vi "read_raw_dataV2.0.vi"() -> ()   [LabVIEW 2017]
uses:
  <vilib>/Utility/file.llb/Read Delimited Spreadsheet (I64).vi
  <vilib>/Utility/file.llb/Write Delimited Spreadsheet (DBL).vi
  <vilib>/Utility/file.llb/Write Delimited Spreadsheet (I64).vi
  <vilib>/Utility/file.llb/Write Delimited Spreadsheet (string).vi
panel:
  in  "col":i32
  in  "file path (dialog if empty)":path=path "G:/tdc/2017/code_density_rom.mem"
  out "size(s)":i32[](array[numeric])=[2048, 128]
  out "Array":u32[][](array[numeric]) format="%x"
  out "cal":u32[][](graph)
  out "x/y":dbl=0.0025
  out "index":i32=556
  out "time":dbl=31675062850000.0 format="%.000f"
  in  "通道数量":i32=128
  out "fine":u64=861 format="%x"
  out "data 5":string
  in  "ch list":u16[](array[numeric])=[0, 1, 2, 3, 4, 5, 6, 7]
  in  "codeDensity":path=path "G:/tdc/2017/test_20240607_060014_codeDensity.csv"
  out "file path (dialog if empty) 2":path=path "G:/tdc/2017/test_20240327_022214.txt"
  out "ip":u64=35 format="%x"
  out "data 9":string="#"
  out "result string":string="test_20240327_022214"
  out "sent number":u64=71 format="%x"
  out "trigger number":u64=71 format="%x"
  out "data 8":string
  out "data 7":string
  out "data":u64[](array[numeric])=[35, 5, 71, 71, 31675062850000] format="%x"
  out "data 2":string
  out "data 4":string
  out "coarse time":u64=12670025140 format="%x"
  out "error out":errorcluster
  out "substring":string="…"
  out "number 3":u32
  out "channel number":u64=5 format="%x"
  in  "channel":u64
  out "data 6":string
  out "data 3":string="Z"
  in  "dat file (use dialog)":path=path "G:/tdc/2017/test_20240607_060014.dat"
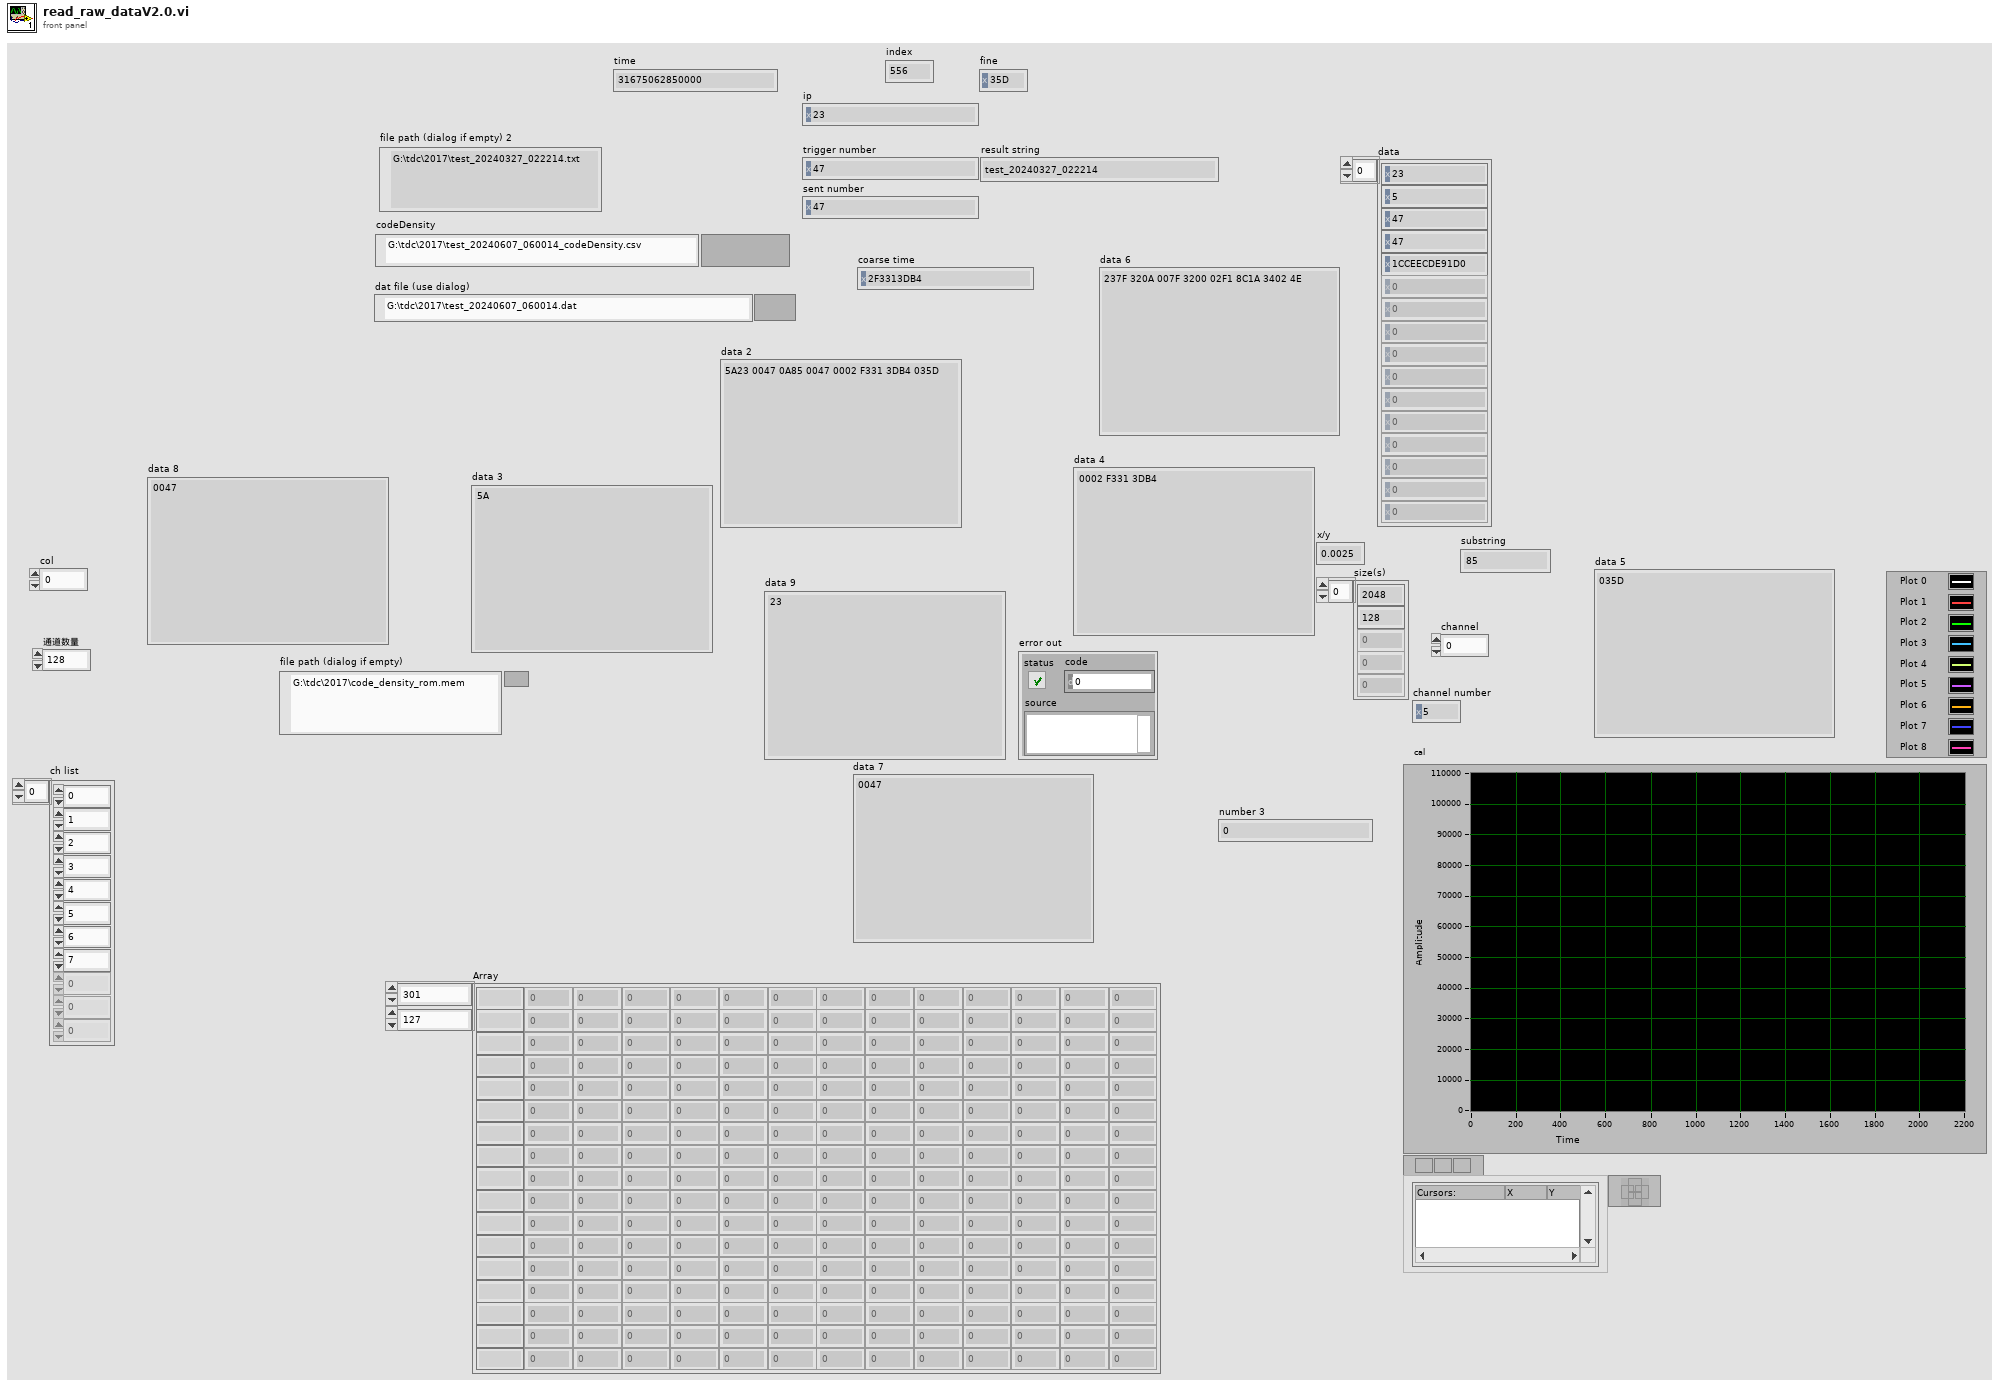
[diagram p1: front panel]
types:
  T1 = enum16{"open", "replace", "create", "open or create", "replace or create", "replace or create with confirmation"}
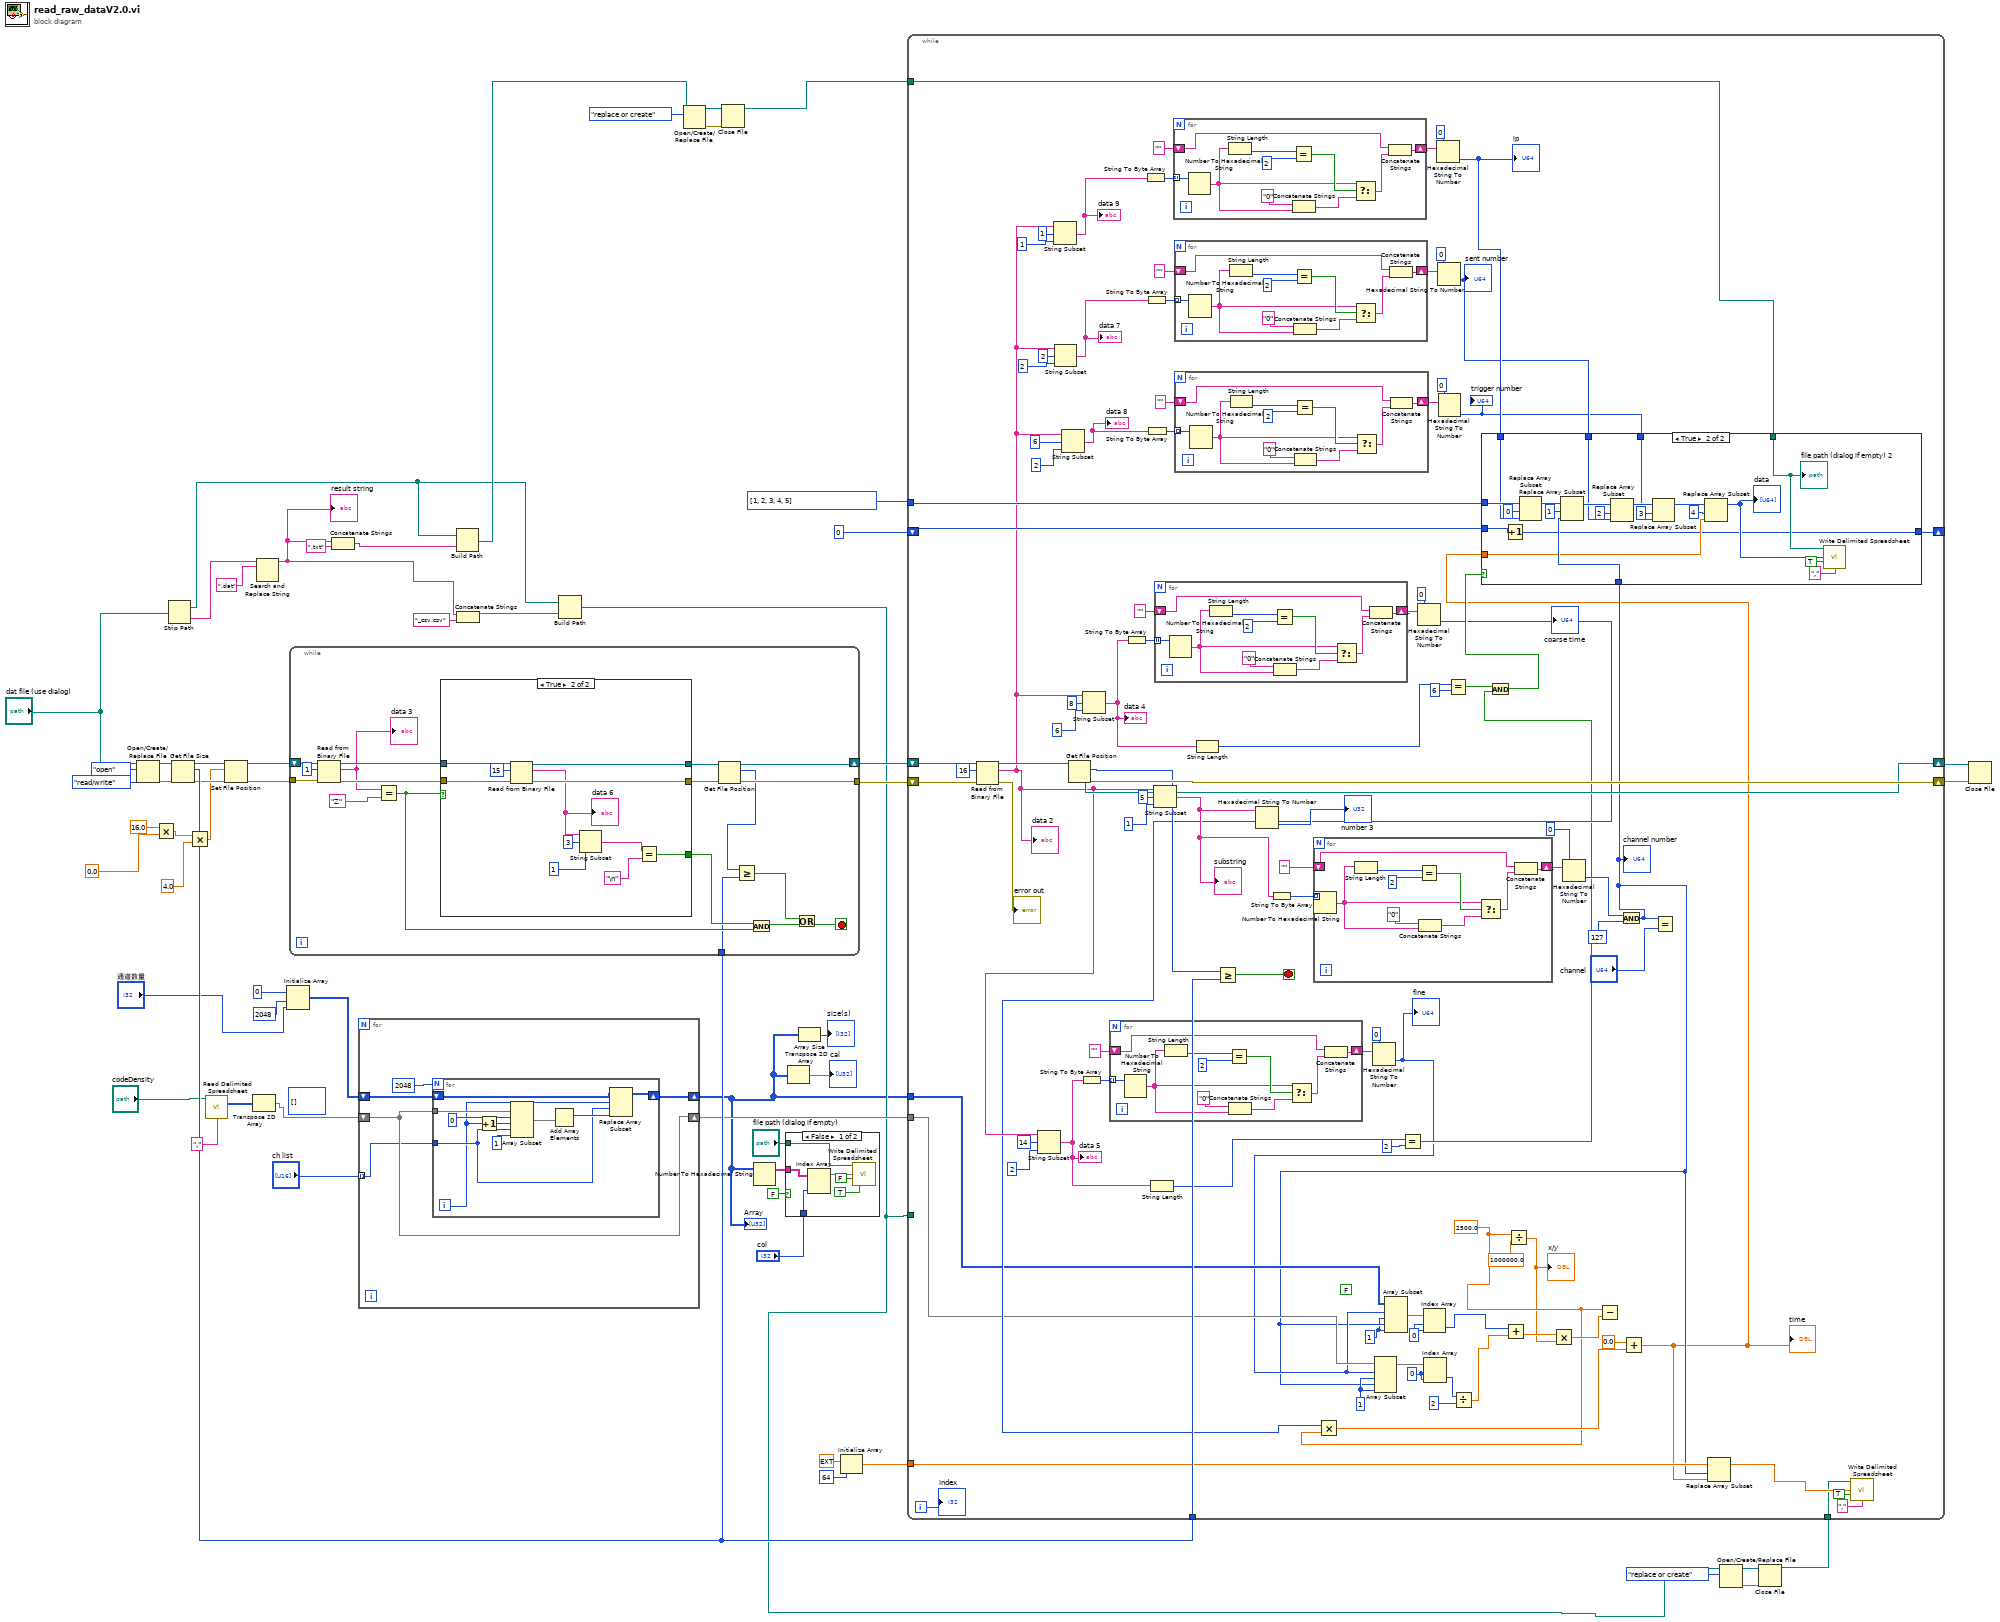
[diagram p0: block diagram]
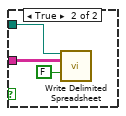
[diagram p2: hidden frame]
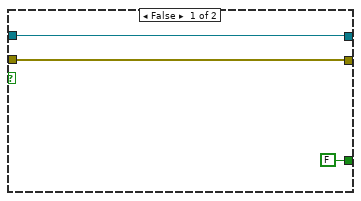
[diagram p4: hidden frame]
diagram:
  (unwired) i64[][] []
  n1 = Open/Create/Replace File(file path (use dialog)="dat file (use dialog)", operation (0:open)=T1."open", access (0:read/write)=enum16{"read/write", "read-only", "write-only"}."read/write") -> (refnum out=w59:refnum<file>, error out=w54:errorcluster)  [unwired: 3 in, 1 out]
  n2 = Multiply(x=16.0, y=0.0) -> (x*y=w20:dbl)
  n3 = Strip Path(path="dat file (use dialog)") -> (stripped path=w9:path, name=w47:string)
  n4 = Get File Size(file=w59, error in=w54) -> (refnum out=w26:refnum<file>, size (in bytes)=w49:i64, 0:w24:errorcluster)
  n5 = Multiply(x=w20, y=4.0) -> (x*y=w18:dbl)
  n6 = call-poly <vilib>:"Read Delimited Spreadsheet.vi"("file path (dialog if empty)"="codeDensity", "delimiter (\\t)"="," ("delimiter (\\t)")) -> ("all rows"=w43:i64[][])  [unwired: 8 in, 5 out]
  n7 = Set File Position(offset (in bytes) (0)=w18, refnum=w26, error in=w24) -> (refnum out=w25:refnum<file>, error out=w23:errorcluster)  [unwired: 1 in]
  n8 = Transpose 2D Array(2D array=w43) -> (transposed array=w31:i64[][])
  n9 = Search and Replace String(input string=w47, search string=".dat") -> (result string=w11:string)  [unwired: 6 in, 3 out]
  "result string" <- w11
  n10 = Initialize Array(u32 0 ("element"), 2048 ("dimension size"), "通道数量") -> (w32:u32[][])
  n11 = while {
    tunnel: w23 -> [w76]
    shift-right: [w64] -> w55
    shift-left: w25 -> [w77]
    tunnel: [w65] -> w56
    tunnel: w49 -> [w63]
    stop <- w61 stop-if-true
    n12 = Read from Binary File(8:w76, 10:1 ("count (1)"), 11:w77) -> (0:w72:errorcluster, 2:w70:string, 3:w73:refnum<file>)  [unwired: 3 in, 1 out]
    "data 3" <- w70
    n13 = Equal?(x=w70, y="Z") -> (x = y?=w67:bool)
    n14 = case shown="True" w67 {
      tunnel: w73 -> [w80 w91]
      tunnel: w72 -> [w79 w90]
      tunnel: [w80 w88] -> w71
      tunnel: [w79 w87] -> w66
      tunnel: [FALSE w81] -> w68
      frame False {
      }
      frame True {
        n15 = Read from Binary File(8:w90, 10:15 ("count (1)"), 11:w91) -> (0:w87:errorcluster, 2:w84:string, 3:w88:refnum<file>)  [unwired: 3 in, 1 out]
        "data 6" <- w84
        n16 = String Subset(string=w84, offset (0)=3, length (rest)=1 ("length (rest)")) -> (substring=w83:string)
        n17 = Equal?(x=w83, y="\n") -> (x = y?=w81:bool)
      }
    }
    n18 = Get File Position(4:w66, 7:w71) -> (0:w65:errorcluster, 2:w62:i64, 3:w64:refnum<file>)
    n19 = Greater Or Equal?(x=w62, y=w63) -> (x >= y?=w60:bool)
    n20 = Compound Arithmetic op=AND(w68, w67) -> (w69:bool)
    n21 = Or(x=w60, y=w69) -> (x .or. y?=w61:bool)
  }
  n22 = Concatenate Strings(w11, ".txt" ("string")) -> (w44:string)
  n23 = for {
    shift-right: [w94] -> w4
    shift-left: w32 -> [w95]
    shift-right: [w93] -> w39
    shift-left: w31 -> [w93]
    tunnel: "ch list" -> [w92] mode=indexing
    n24 = for {
      N: 2048 -> [_]
      tunnel: w93 -> [w106]
      tunnel: w92 -> [w99]
      shift-right: [w101] -> w94
      shift-left: w95 -> [w102]
      i -> [w98]
      n25 = Increment(x=w98) -> (x+1=w97:i32)
      n26 = Array Subset(array=w106, index (row)=0 ("索引"), length (row)=w97, index (col)=w99, length (col)=1 ("长度")) -> (w103:i64[][])
      n27 = Add Array Elements(numeric array=w103) -> (sum=w100:i64)
      n28 = Replace Array Subset(array=w102, new element=w100, index (row)=w98, index (col)=w99) -> (w101:u32[][])
    }
  }
  "Array" <- w4
  n29 = Build Path(base path=w9, name or relative path=w44) -> (appended path=w14:path)
  n30 = Concatenate Strings(w11, "_csv.csv" ("string")) -> (w10:string)
  n31 = Build Path(base path=w9, name or relative path=w10) -> (appended path=w8:path)
  n32 = Open/Create/Replace File(file path (use dialog)=w14, operation (0:open)=T1."replace or create") -> (refnum out=w15:refnum<file>, error out=w16:errorcluster)  [unwired: 4 in, 1 out]
  n33 = Close File(refnum=w15, error in=w16) -> (path=w13:path)  [unwired: 1 out]
  n34 = Number To Hexadecimal String(2:w4) -> (0:w3:string[][])  [unwired: 1 in]
  n35 = case shown="False" FALSE {
    tunnel: "file path (dialog if empty)" -> [w111 w115]
    tunnel: w3 -> [w110 w113]
    tunnel: "col" -> [w108 _]
    frame False {
      n36 = Index Array(array=w110, index (col)=w108) -> (element=w109:string[])  [unwired: 1 in]
      n37 = call-poly <vilib>:"Write Delimited Spreadsheet.vi"("file path (dialog if empty)"=w111, "1D data"=w109, "append to file? (new file:F)"=FALSE, "transpose? (no:F)"=TRUE) -> ()  [unwired: 10 in, 2 out]
    }
    frame True {
      n38 = call-poly <vilib>:"Write Delimited Spreadsheet.vi"("file path (dialog if empty)"=w115, "2D data"=w113, "append to file? (new file:F)"=FALSE) -> ()  [unwired: 11 in, 2 out]
    }
  }
  n39 = Transpose 2D Array(2D array=w4) -> (transposed array=→"cal":u32[][])
  n40 = Array Size(array=w4) -> (size(s)=→"size(s)":i32[])
  n41 = Initialize Array(ext 0.0 ("element"), 64 ("dimension size")) -> (w36:ext[])
  n42 = Open/Create/Replace File(file path (use dialog)=w8, operation (0:open)=T1."replace or create") -> (refnum out=w28:refnum<file>, error out=w29:errorcluster)  [unwired: 4 in, 1 out]
  n43 = Close File(refnum=w28, error in=w29) -> (path=w27:path)  [unwired: 1 out]
  n44 = while {
    shift-right: [w210] -> w53
    shift-left: w55 -> [w214]
    shift-right: [w212] -> w52
    shift-left: w56 -> [w215]
    tunnel: w49 -> [w208]
    shift-right: [w156] -> _
    shift-left: 0 ("length (rest)") -> [w187]
    tunnel: w13 -> [w157]
    tunnel: u64[] [1, 2, 3, 4, 5] -> [w186]
    tunnel: w4 -> [w130]
    tunnel: w39 -> [w131]
    tunnel: w36 -> [w126]
    tunnel: w27 -> [w118]
    tunnel: w8 -> [_]
    i -> [w117]
    stop <- w207 stop-if-true
    w119 = 0 ("index (row)")
    w121 = 1 ("长度")
    w133 = 2500.0 ("x")
    (unwired) FALSE
    w147 = 0 ("索引 (行)")
    w149 = 1 ("长度")
    n45 = Read from Binary File(8:w215, 10:16 ("count (1)"), 11:w214) -> (0:→"error out":errorcluster, 2:w135:string, 3:w211:refnum<file>)  [unwired: 3 in, 1 out]
    "data 2" <- w135
    n46 = String Subset(string=w135, offset (0)=14, length (rest)=2 ("length (rest)")) -> (substring=w138:string)
    "data 5" <- w138
    n47 = String Subset(string=w135, offset (0)=1, length (rest)=1 ("length (rest)")) -> (substring=w167:string)
    "data 9" <- w167
    n48 = String Subset(string=w135, offset (0)=2, length (rest)=2 ("length (rest)")) -> (substring=w168:string)
    "data 7" <- w168
    n49 = String Subset(string=w135, offset (0)=6, length (rest)=2 ("length (rest)")) -> (substring=w173:string)
    "data 8" <- w173
    n50 = Get File Position(7:w211) -> (0:w212:errorcluster, 2:w209:i64, 3:w210:refnum<file>)  [unwired: 1 in]
    n51 = String To Byte Array(string=w138) -> (unsigned byte array=w141:u8[])
    n52 = String Subset(string=w135, offset (0)=8, length (rest)=6 ("length (rest)")) -> (substring=w184:string)
    "data 4" <- w184
    n53 = for {
      shift-right: [w224] -> w140
      shift-left: "" ("format string") -> [w221]
      tunnel: w141 -> [w225] mode=indexing
      n54 = Number To Hexadecimal String(2:w225) -> (0:w217:string)  [unwired: 1 in]
      n55 = String Length(string=w217) -> (length=w223:i32)
      n56 = Equal?(x=w223, y=2) -> (x = y?=w220:bool)
      n57 = Concatenate Strings("0" ("format string"), w217) -> (w219:string)
      n58 = Select(t=w217, s=w220, f=w219) -> (s? t:f=w216:string)
      n59 = Concatenate Strings(w221, w216) -> (w224:string)
    }
    n60 = String To Byte Array(string=w184) -> (unsigned byte array=w203:u8[])
    n61 = String To Byte Array(string=w167) -> (unsigned byte array=w164:u8[])
    n62 = String To Byte Array(string=w168) -> (unsigned byte array=w171:u8[])
    n63 = String To Byte Array(string=w173) -> (unsigned byte array=w175:u8[])
    n64 = String Length(string=w138) -> (length=w137:i32)
    n65 = String Subset(string=w135, offset (0)=5, length (rest)=1 ("length (rest)")) -> (substring=w190:string)
    "substring" <- w190
    n66 = for {
      shift-right: [w296] -> w202
      shift-left: "" ("format string") -> [w293]
      tunnel: w203 -> [w297] mode=indexing
      n67 = Number To Hexadecimal String(2:w297) -> (0:w289:string)  [unwired: 1 in]
      n68 = String Length(string=w289) -> (length=w295:i32)
      n69 = Equal?(x=w295, y=2) -> (x = y?=w292:bool)
      n70 = Concatenate Strings("0" ("format string"), w289) -> (w291:string)
      n71 = Select(t=w289, s=w292, f=w291) -> (s? t:f=w288:string)
      n72 = Concatenate Strings(w293, w288) -> (w296:string)
    }
    n73 = for {
      shift-right: [w234] -> w165
      shift-left: "" ("format string") -> [w231]
      tunnel: w164 -> [w235] mode=indexing
      n74 = Number To Hexadecimal String(2:w235) -> (0:w227:string)  [unwired: 1 in]
      n75 = String Length(string=w227) -> (length=w233:i32)
      n76 = Equal?(x=w233, y=2) -> (x = y?=w230:bool)
      n77 = Concatenate Strings("0" ("format string"), w227) -> (w229:string)
      n78 = Select(t=w227, s=w230, f=w229) -> (s? t:f=w226:string)
      n79 = Concatenate Strings(w231, w226) -> (w234:string)
    }
    n80 = for {
      shift-right: [w244] -> w170
      shift-left: "" ("format string") -> [w241]
      tunnel: w171 -> [w245] mode=indexing
      n81 = Number To Hexadecimal String(2:w245) -> (0:w237:string)  [unwired: 1 in]
      n82 = String Length(string=w237) -> (length=w243:i32)
      n83 = Equal?(x=w243, y=2) -> (x = y?=w240:bool)
      n84 = Concatenate Strings("0" ("format string"), w237) -> (w239:string)
      n85 = Select(t=w237, s=w240, f=w239) -> (s? t:f=w236:string)
      n86 = Concatenate Strings(w241, w236) -> (w244:string)
    }
    n87 = for {
      shift-right: [w254] -> w176
      shift-left: "" ("format string") -> [w251]
      tunnel: w175 -> [w255] mode=indexing
      n88 = Number To Hexadecimal String(2:w255) -> (0:w247:string)  [unwired: 1 in]
      n89 = String Length(string=w247) -> (length=w253:i32)
      n90 = Equal?(x=w253, y=2) -> (x = y?=w250:bool)
      n91 = Concatenate Strings("0" ("format string"), w247) -> (w249:string)
      n92 = Select(t=w247, s=w250, f=w249) -> (s? t:f=w246:string)
      n93 = Concatenate Strings(w251, w246) -> (w254:string)
    }
    n94 = String Length(string=w184) -> (length=w182:i32)
    n95 = Greater Or Equal?(x=w209, y=w208) -> (x >= y?=w207:bool)
    n96 = Hexadecimal String To Number(string=w190) -> (number=→"number 3":u32)  [unwired: 2 in, 1 out]
    n97 = String To Byte Array(string=w190) -> (unsigned byte array=w193:u8[])
    n98 = for {
      shift-right: [w286] -> w192
      shift-left: "" ("format string") -> [w283]
      tunnel: w193 -> [w287] mode=indexing
      n99 = Number To Hexadecimal String(2:w287) -> (0:w279:string)  [unwired: 1 in]
      n100 = String Length(string=w279) -> (length=w285:i32)
      n101 = Equal?(x=w285, y=2) -> (x = y?=w282:bool)
      n102 = Concatenate Strings("0" ("format string"), w279) -> (w281:string)
      n103 = Select(t=w279, s=w282, f=w281) -> (s? t:f=w278:string)
      n104 = Concatenate Strings(w283, w278) -> (w286:string)
    }
    n105 = Hexadecimal String To Number(string=w140, default (0uL)=u64 0 ("default (0 U32)")) -> (number=w128:u64)  [unwired: 1 in, 1 out]
    "fine" <- w128
    n106 = Equal?(x=w137, y=2) -> (x = y?=w129:bool)
    n107 = Hexadecimal String To Number(string=w202, default (0uL)=u64 0 ("default (0 U32)")) -> (number=w134:u64)  [unwired: 1 in, 1 out]
    "coarse time" <- w134
    n108 = Multiply(x=w134, y=w133) -> (x*y=w151:dbl)
    n109 = Hexadecimal String To Number(string=w165, default (0uL)=u64 0 ("default (0 U32)")) -> (number=w160:u64)  [unwired: 1 in, 1 out]
    "ip" <- w160
    n110 = Hexadecimal String To Number(string=w170, default (0uL)=u64 0 ("default (0 U32)")) -> (number=w159:u64)  [unwired: 1 in, 1 out]
    "sent number" <- w159
    n111 = Hexadecimal String To Number(string=w176, default (0uL)=u64 0 ("default (0 U32)")) -> (number=w158:u64)  [unwired: 1 in, 1 out]
    "trigger number" <- w158
    n112 = Equal?(x=w182, y=6) -> (x = y?=w183:bool)
    n113 = And(x=w183, y=w129) -> (x .and. y?=w180:bool)
    n114 = Divide(x=w133, y=1000000.0) -> (x/y=w132:dbl)
    "x/y" <- w132
    n115 = Hexadecimal String To Number(string=w192, default (0uL)=u64 0 ("default (0 U32)")) -> (number=w189:u64)  [unwired: 1 in, 1 out]
    n116 = And(x=w189, y=u64 127 ("default (0 U32)")) -> (x .and. y?=w125:u64)
    "channel number" <- w125
    n117 = Array Subset(array=w131, index (row)=w128, length (row)=w149, index (col)=w125, length (col)=w149) -> (w148:i64[][])
    n118 = Array Subset(array=w130, index (row)=w128, length (row)=w121, index (col)=w125, length (col)=w121) -> (w120:u32[][])
    n119 = Index Array(array=w120, index (row)=w119, index (col)=w119) -> (element=w153:u32)
    n120 = Index Array(array=w148, index (row)=w147, index (col)=w147) -> (element=w146:i64)
    n121 = Divide(x=w146, y=u32 2) -> (x/y=w150:dbl)
    n122 = Add(x=w153, y=w150) -> (x+y=w152:dbl)
    n123 = Multiply(x=w152, y=w132) -> (x*y=w145:dbl)
    n124 = Subtract(x=w133, y=w145) -> ()  [unwired: 1 out]
    n125 = Add(x=0.0, y=w151) -> (x+y=w124:dbl)
    "time" <- w124
    n126 = case shown="True" w180 {
      tunnel: w187 -> [w256 w259]
      tunnel: w186 -> [_ w277]
      tunnel: w124 -> [_ w260]
      tunnel: w160 -> [_ w275]
      tunnel: w159 -> [_ w267]
      tunnel: w158 -> [_ w268]
      tunnel: w125 -> [_ w266]
      tunnel: w157 -> [_ w264]
      tunnel: [w256 w258] -> w156
      frame False {
      }
      frame True {
        n127 = Increment(x=w259) -> (x+1=w258:i32)
        n128 = Replace Array Subset(array=w277, new element=w275, index=0) -> (w274:u64[])
        n129 = Replace Array Subset(array=w274, new element=w266, index=1) -> (w269:u64[])
        n130 = Replace Array Subset(array=w269, new element=w267, index=2) -> (w271:u64[])
        n131 = Replace Array Subset(array=w271, new element=w268, index=3) -> (w262:u64[])
        n132 = Replace Array Subset(array=w262, new element=w260, index=4) -> (w261:u64[])
        "data" <- w261
        n133 = call-poly <vilib>:"Write Delimited Spreadsheet.vi"("file path (dialog if empty)"=w264, "1D data"=w261, "append to file? (new file:F)"=TRUE, "delimiter (\\t)"="," ("delimiter (\\t)")) -> ()  [unwired: 10 in, 2 out]
        "file path (dialog if empty) 2" <- w264
      }
    }
    n134 = Equal?(x=w125, y="channel") -> ()  [unwired: 1 out]
    n135 = Replace Array Subset(array=w126, new element=w124, index=w125) -> (w123:ext[])
    n136 = call-poly <vilib>:"Write Delimited Spreadsheet.vi"("file path (dialog if empty)"=w118, "1D data"=w123, "append to file? (new file:F)"=TRUE, "delimiter (\\t)"="," ("delimiter (\\t)")) -> ()  [unwired: 10 in, 2 out]
    "index" <- w117
  }
  n137 = Close File(refnum=w53, error in=w52) -> ()  [unwired: 2 out]
